vi "Image_Folder.vi"(8 "New":i32, 9 "Old":i32, 10 "Other":i32, 11 "input cluster":T1={"L16 Linear Actuator"="", "XE 1000 Pump"="", "Camera1"="", "Camera2"="", "Camera1_IMG"=refnum, "Camera2_IMG"=refnum, "Img_Capt"=FALSE, "Actuator"=FALSE, "Pump"=FALSE, "Cam 1"=FALSE, "Cam 2"=FALSE, "Empty_Refill"=FALSE, "Crop"=FALSE, "Light intensity"=100, "Exposure Time"=1000.0, "Sample Name"="Test Sample", "Operator"="MRJ", "Calibration 1"=path "C:/Users/au540322/Desktop/IHS_Project/images/Debris/Debris_0/Debris_0_2019_06_01-23-32-49-686.PNG", "Calibration 2"=path "C:/Users/au540322/Desktop/IHS_Project/images/Debris/Debris_0/Debris_0_2019_06_01-23-32-49-686.PNG", "Framerate"=1, "Timeout Sample"=50, "Collection date"="MRJ", "Sample size threshold"=1, "Empty start"=1, "Command"="MRJ", "Calibration Image 1"=refnum, "Calibration Image 2"=refnum, "Original Image 1"=refnum, "Original Image 2"=refnum, "Processing Image 1"=refnum, "Processing Image 2"=refnum, "Object Image 1"=refnum, "Object Image 2"=refnum, "Cam 1 - save queue"=refnum, "Cam 2 - save queue"=refnum, "Station"="", "Species Name"="", "Other Notes"="", "Aperture"=enum."Item 0", "Image Process Queue Size"=500, "Image Save Queue Size"=500, "Overload threshold"=500, "Max Framerate"=100, "Blue Plane Image"=refnum, "Subtract Image"=refnum, "Binary Image 1"=refnum, "ROI mask allocation"=refnum, "Rectangle 1"={"Left"=0, "Top"=0, "Right"=0, "Bottom"=0, "Rotation"=0.0}, "Rectangle 2"={"Left"=0, "Top"=0, "Right"=0, "Bottom"=0, "Rotation"=0.0}, "Binary Image 2"=refnum, "Detection Region %"=0.0, "Cam 1 queue"=refnum, "Cam 2 queue"=refnum, "Detect image 1"=refnum, "Detect image 2"=refnum, "Detect 1"=path "C:/Users/au540322/Desktop/IHS_Project/images/Debris/Debris_0/Debris_0_2019_06_01-23-32-49-686.PNG", "Detect 2"=path "C:/Users/au540322/Desktop/IHS_Project/images/Debris/Debris_0/Debris_0_2019_06_01-23-32-49-686.PNG", "Max large object threshold"=0, "Open(T)/Close(F)"=FALSE} {"Rectangle 2"."Rotation" format="%.2f"; "Rectangle 2"."Left" scale=0.0..1024.0; "Rectangle 2"."Right" scale=0.0..1024.0; "Rectangle 1"."Rotation" format="%.2f"; "Rectangle 1"."Left" scale=0.0..1024.0; "Rectangle 1"."Right" scale=0.0..1024.0; "Max Framerate" min=1; "Overload threshold" min=1; "Image Save Queue Size" min=1; "Image Process Queue Size" min=1; "Empty start" min=1; "Sample size threshold" min=1; "Framerate" min=1; "Light intensity" scale=0.0..100.0}) -> (2 "Subfolder Name":string, 3 "Subfolder Path":string)   [LabVIEW 2019]
uses:
  controls/Data.ctl
  <vilib>/userdefined/High Color/IMAQdx.ctl
  <vilib>/vision/Image Controls.llb/IMAQ Image.ctl
panel:
  out "error out 2":errorcluster
  out "error out":errorcluster
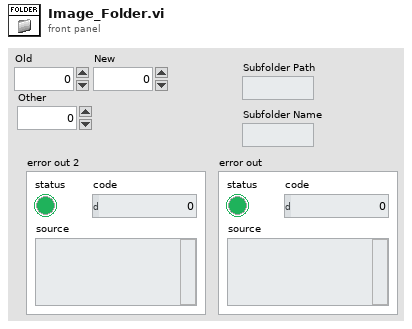
[diagram p1: front panel]
types:
  T1 = typedef "Data.ctl" = cluster{"L16 Linear Actuator":refnum<visa-resource-name>, "XE 1000 Pump":refnum<visa-resource-name>, "Camera1":T2, "Camera2":T2, "Camera1_IMG":T3, "Camera2_IMG":T3, "Img_Capt":bool, "Actuator":bool, "Pump":bool, "Cam 1":bool, "Cam 2":bool, "Empty_Refill":bool, "Crop":bool, "Light intensity":i32, "Exposure Time":dbl, "Sample Name":string, "Operator":string, "Calibration 1":path, "Calibration 2":path, "Framerate":i32, "Timeout Sample":i32, "Collection date":string, "Sample size threshold":i32, "Empty start":u32, "Command":string, "Calibration Image 1":T3, "Calibration Image 2":T3, "Original Image 1":T3, "Original Image 2":T3, "Processing Image 1":T3, "Processing Image 2":T3, "Object Image 1":T3, "Object Image 2":T3, "Cam 1 - save queue":refnum<queue>, "Cam 2 - save queue":refnum<queue>, "Station":string, "Species Name":string, "Other Notes":string, "Aperture":enum32{"Item 0", "Item 1", "Item 2", "Item 3"}, "Image Process Queue Size":i32, "Image Save Queue Size":i32, "Overload threshold":i32, "Max Framerate":i32, "Blue Plane Image":T3, "Subtract Image":T3, "Binary Image 1":T3, "ROI mask allocation":T3, "Rectangle 1":T4, "Rectangle 2":T4, "Binary Image 2":T3, "Detection Region %":dbl, "Cam 1 queue":refnum<queue>, "Cam 2 queue":refnum<queue>, "Detect image 1":T3, "Detect image 2":T3, "Detect 1":path, "Detect 2":path, "Max large object threshold":i32, "Open(T)/Close(F)":bool}
  T2 = typedef "IMAQdx.ctl" = refnum<k21>
  T3 = typedef "IMAQ Image.ctl" = refnum<image>
  T4 = typedef "IMAQ Rectangle" = cluster{"Left":i32, "Top":i32, "Right":i32, "Bottom":i32, "Rotation":dbl}
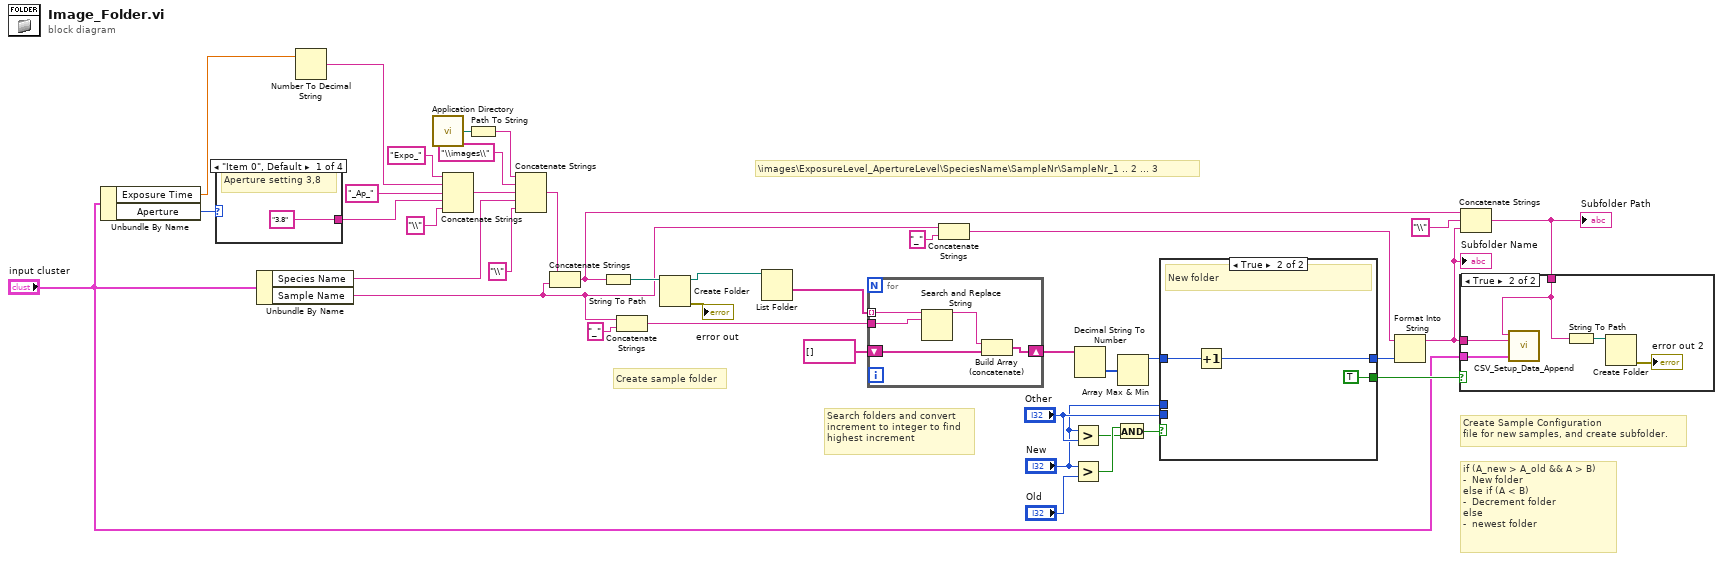
[diagram p0: block diagram]
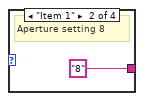
[diagram p2: hidden frame]
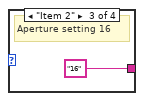
[diagram p3: hidden frame]
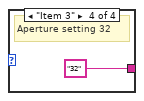
[diagram p4: hidden frame]
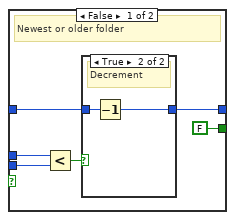
[diagram p5: hidden frame]
diagram:
  # "\\images\\ExposureLevel_ApertureLevel\\SpeciesName\\SampleNr\\SampleNr_1 .. 2 ... 3"
  # "if (A_new > A_old && A > B)\n-  New folder\nelse if (A < B)\n-  Decrement folder\nelse \n-  newest folder"
  # "Create Sample Configuration \nfile for new samples, and create subfolder."
  # "Search folders and convert \nincrement to integer to find\nhighest increment"
  # "Create sample folder"
  n1 = Unbundle By Name("input cluster") -> ("Exposure Time"=w9:dbl, "Aperture"=w6:enum32{"Item 0", "Item 1", "Item 2", "Item 3"})
  n2 = case shown="\"Item 0\", Default" w6 {
    tunnel: ["3.8" "8" "16" "32"] -> w3
    frame "Item 0", Default {
      # "Aperture setting 3,8"
    }
    frame "Item 1" {
      # "Aperture setting 8"
    }
    frame "Item 2" {
      # "Aperture setting 16"
    }
    frame "Item 3" {
      # "Aperture setting 32"
    }
  }
  n3 = Unbundle By Name("input cluster") -> ("Species Name"=w14:string, "Sample Name"=w12:string)
  n4 = Number To Decimal String(number=w9) -> (decimal integer string=w4:string)  [unwired: 1 in]
  n5 = call <vilib>:"Application Directory.vi"() -> ("Application Directory"=w33:path)
  n6 = Concatenate Strings("Expo_" ("string"), w4, "_Ap_" ("string"), w3, "\\" ("string")) -> (w1:string)
  n7 = Path To String(path=w33) -> (string=w34:string)
  n8 = Concatenate Strings(w34, "\\images\\" ("string"), w1, w14, "\\" ("string")) -> (w13:string)
  n9 = Concatenate Strings(w13, w12) -> (w11:string)
  n10 = String To Path(string=w11) -> (path=w36:path)
  n11 = Concatenate Strings(w12, "_" ("string")) -> (w31:string)
  n12 = Create Folder(path (use dialog)=w36) -> (created path=w39:path, error out=→"error out":errorcluster)  [unwired: 2 in, 1 out]
  n13 = List Folder(path=w39) -> (folder names=w32:string[])  [unwired: 3 in, 3 out]
  n14 = for {
    tunnel: w32 -> [w49] mode=indexing
    tunnel: w31 -> [w48]
    shift-right: [w46] -> w29
    shift-left: string[] [] -> [w45]
    n15 = Search and Replace String(input string=w49, search string=w48) -> (result string=w47:string)  [unwired: 6 in, 3 out]
    n16 = Build Array (concatenate)(w47, w45) -> (w46:string[])
  }
  n17 = Concatenate Strings(w12, "_" ("string")) -> (w25:string)
  n18 = Greater?(x="New", y="Other") -> (0:w22:bool)
  n19 = Greater?(x="New", y="Old") -> (0:w23:bool)
  n20 = Decimal String To Number(string=w29) -> (number=w28:i32[])  [unwired: 2 in, 1 out]
  n21 = And(x=w23, y=w22) -> (x .and. y?=w21:bool)
  n22 = Array Max & Min(array=w28) -> (max value=w17:i32)  [unwired: 3 out]
  n23 = case shown="True" w21 {
    tunnel: "Other" -> [w55 _]
    tunnel: "New" -> [w54 _]
    tunnel: [FALSE ("New sample (F)") TRUE ("New sample (F)")] -> w18
    tunnel: w17 -> [w52 w60]
    tunnel: [w51 w59] -> w16
    frame False {
      # "Newest or older folder"
      n24 = Less?(x=w54, y=w55) -> (x < y?=w53:bool)
      n25 = case shown="True" w53 {
        tunnel: w52 -> [w56 w58]
        tunnel: [w56 w57] -> w51
        frame False {
          # "Newest folder"
        }
        frame True {
          # "Decrement"
          n26 = Decrement(x=w58) -> (x-1=w57:i32)
        }
      }
    }
    frame True {
      # "New folder"
      n27 = Increment(x=w60) -> (x+1=w59:i32)
    }
  }
  n28 = Format Into String(initial string=w25, w16) -> (resulting string=w26:string)  [unwired: 2 in, 1 out]
  "Subfolder Name" <- w26
  n29 = Concatenate Strings(w11, "\\" ("string"), w26) -> (w15:string)
  "Subfolder Path" <- w15
  n30 = case shown="True" w18 {
    tunnel: w26 -> [_ w63]
    tunnel: "input cluster" -> [_ w62]
    tunnel: w15 -> [_ w64]
    frame False {
    }
    frame True {
      n31 = call "CSV_Setup_Data_Append.vi"("input cluster"=w62, "Sample Name"=w63, "Image path"=w64) -> ()  [unwired: 9 in]
      n32 = String To Path(string=w64) -> (path=w65:path)
      n33 = Create Folder(path (use dialog)=w65) -> (error out=→"error out 2":errorcluster)  [unwired: 2 in, 2 out]
    }
  }
